vi "WeaponChanged_glob.vi"() -> ()   [LabVIEW 2021]
panel:
  out "Boolean":bool
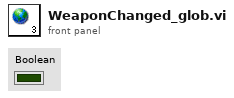
[diagram p1: front panel]
diagram:
